vi "move_to.vi"(2 "error in (no error)":errorcluster caption="错误输入（无错误）", 3 "init? (T)":bool=TRUE, 4 "target pos":dbl, 5 "OneMotion 输入":refnum<class "OneMotion.lvclass">) -> (0 "error out":errorcluster caption="错误输出", 1 "OneMotion 输出":refnum<class "OneMotion.lvclass">)   [LabVIEW 2016, in "MotionControl_UFO_3DOF.lvlib" / "OneMotion.lvclass"]
uses:
  <userlib>/MotionControl_UFO_3DOF/OneMotion/OneMotion.lvclass
  <userlib>/MotionControl_UFO_3DOF/OneMotion/OneMotion.lvclass/OneMotion.ctl
  <userlib>/MotionControl_UFO_3DOF/OneMotion/cmd_motion.ctl
  <userlib>/MotionControl_UFO_3DOF/StepMotor/StepMotor.lvclass
  <userlib>/MotionControl_UFO_3DOF/MotionControl_UFO_3DOF.lvlib
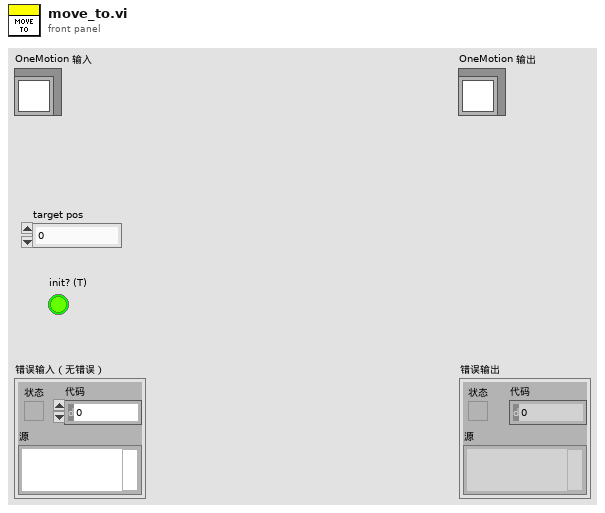
[diagram p1: front panel]
types:
  T1 = cluster{"CAN node ID":i32, "target pos":dbl, "name":string}
  T2 = typedef "MotionControl_UFO_3DOF.lvlib/OneMotion.lvclass/cmd_motion.ctl" = enum16{"NONE", "MOVE_MOTION", "EXIT", "STP_MOTION", "SPEED_MOTION", "WAIT_FOR_S3", "WAIT_A_TIME", "SKIP", "RETRACT_BEFORE_ROT"}
  T3 = cluster{"cmd":T2, cluster{"CAN node ID":i32, "target pos":dbl, "name":string}}
  T4 = cluster{"cmd":T2, cluster{"CAN node ID":i32, "target pos":dbl, "name":string}}[]
  T5 = typedef "MotionControl_UFO_3DOF.lvlib/OneMotion.lvclass/backlash option.ctl" = enum16{"no backlash compensation", "compensation: from - to +", "compensation: from + to -"}
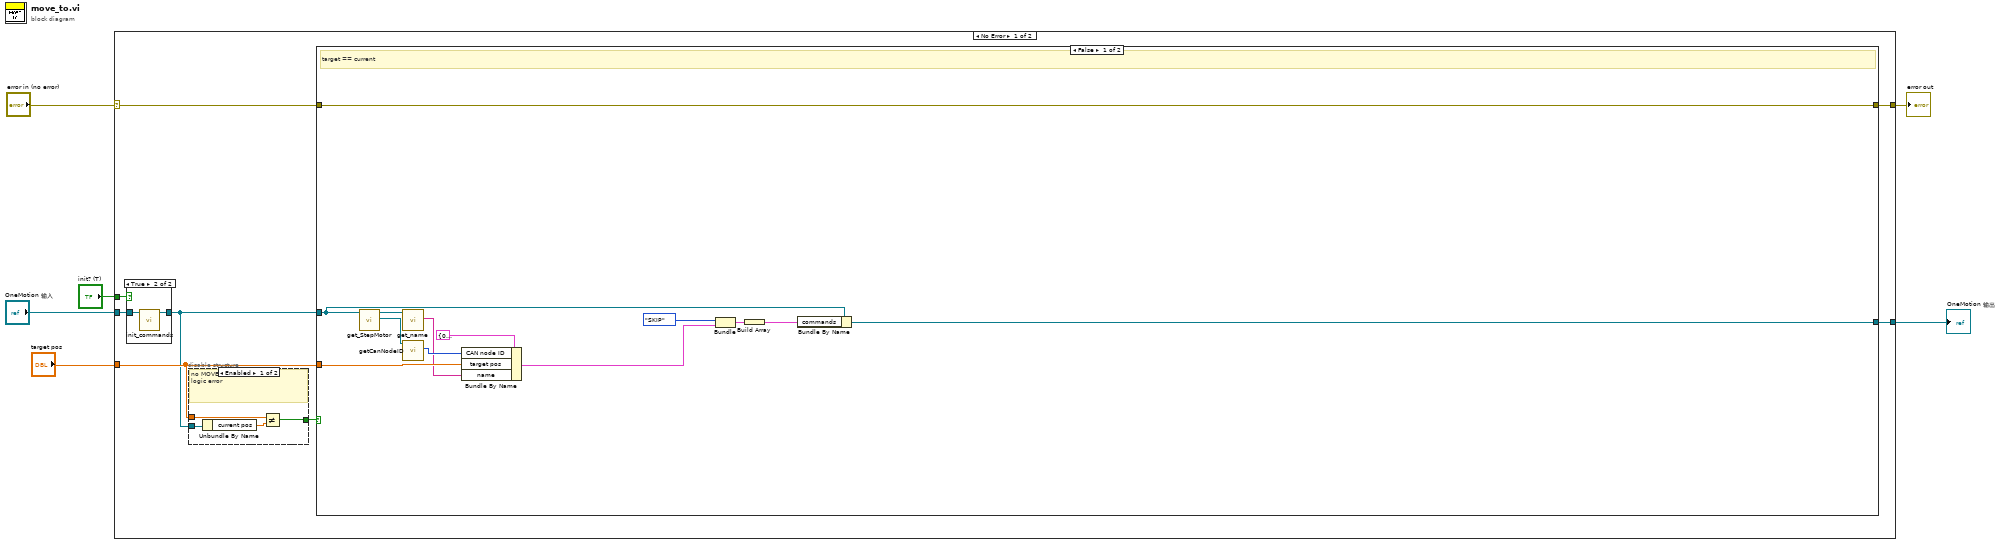
[diagram p0: block diagram]
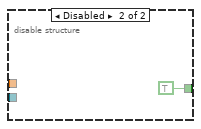
[diagram p2: hidden frame]
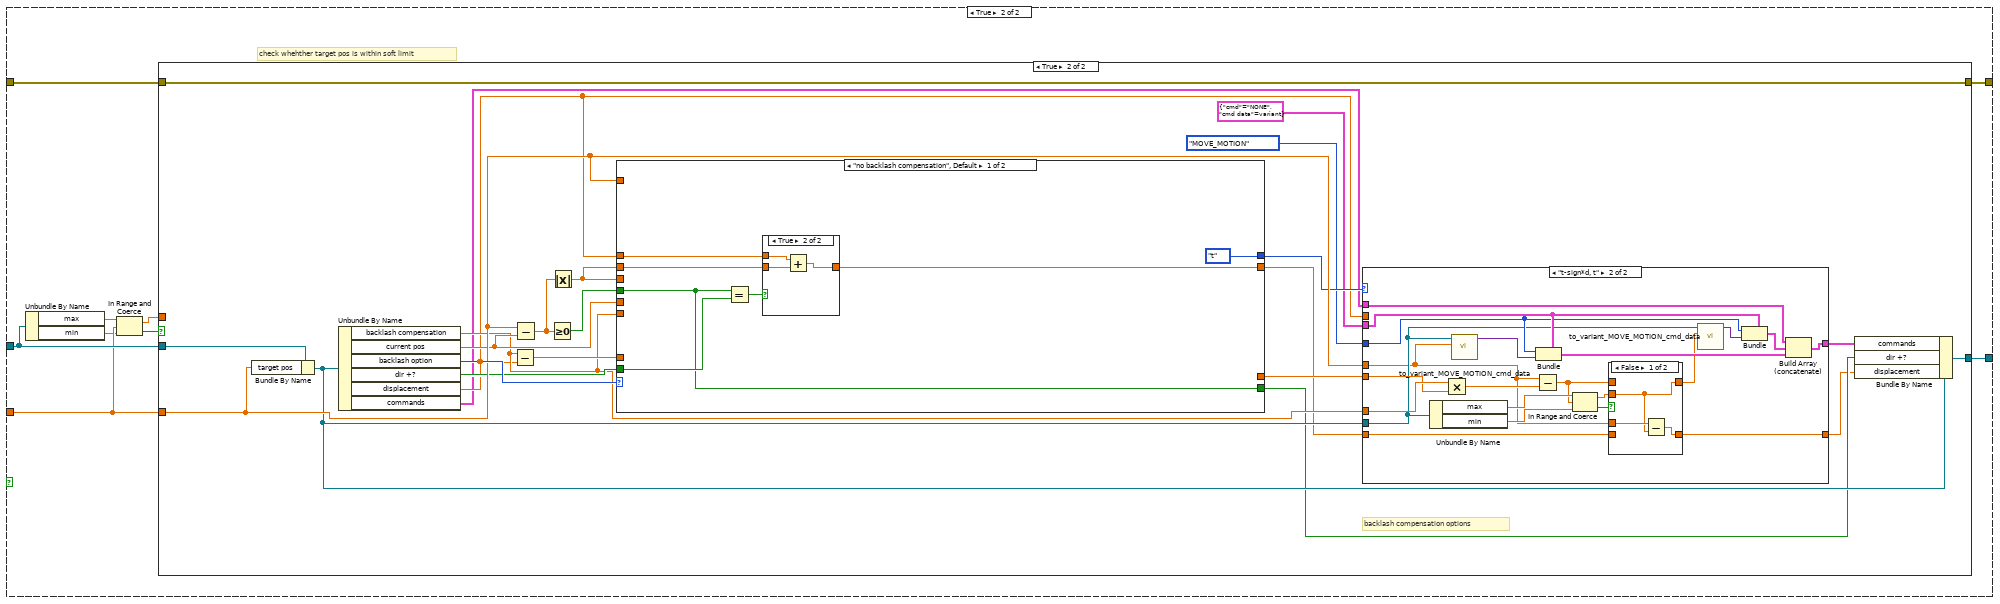
[diagram p4: hidden frame]
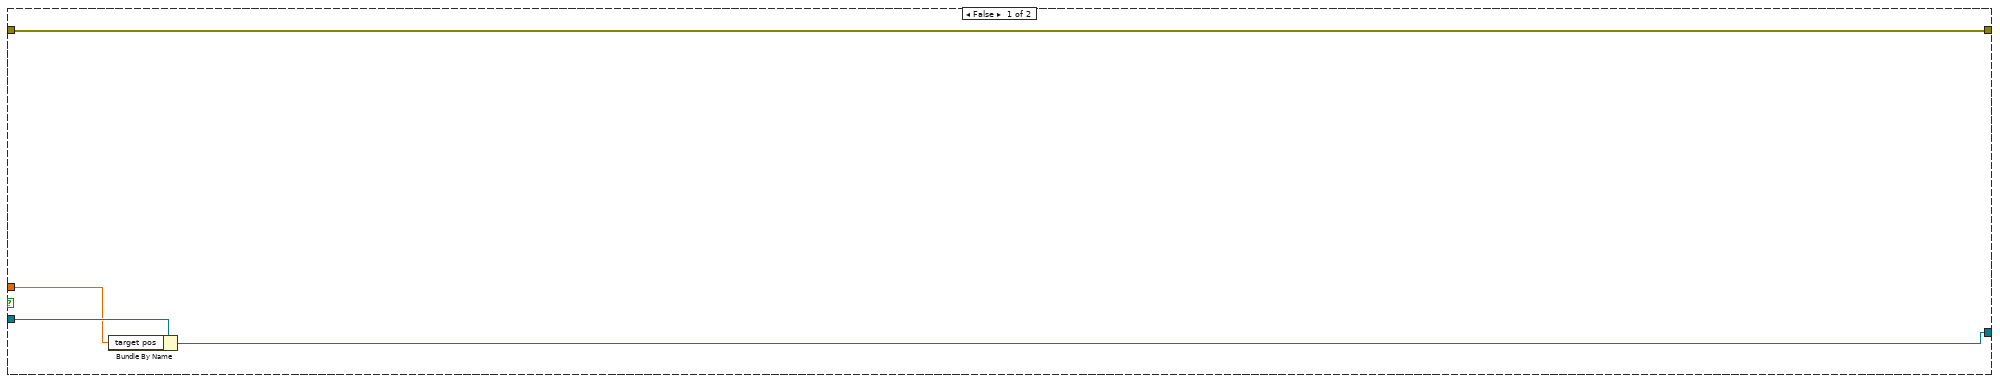
[diagram p5: hidden frame]
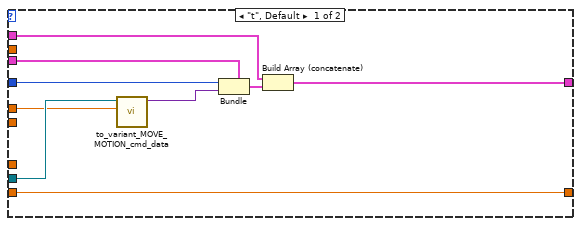
[diagram p6: hidden frame]
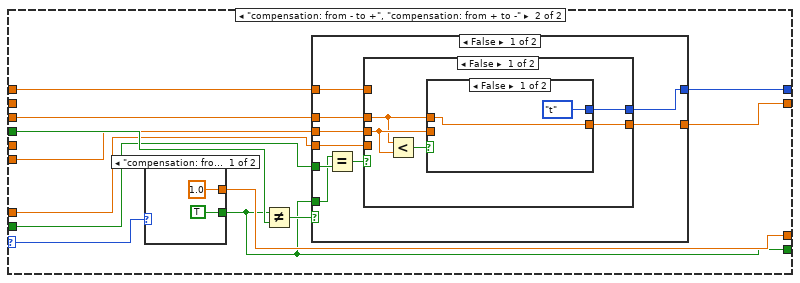
[diagram p9: hidden frame]
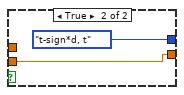
[diagram p10: hidden frame]
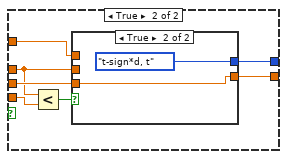
[diagram p11: hidden frame]
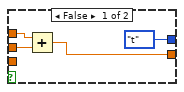
[diagram p12: hidden frame]
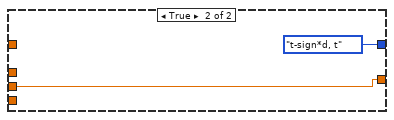
[diagram p13: hidden frame]
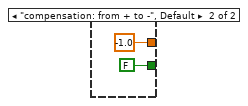
[diagram p14: hidden frame]
diagram:
  n1 = case shown="No Error" "error in (no error)" {
    selector: "error in (no error)" -> [w13 w168]
    tunnel: [w12 w168] -> w5
    tunnel: [w14 w167] -> w4
    tunnel: "OneMotion 输入" -> [w8 w167]
    tunnel: "target pos" -> [w11 _]
    tunnel: "init? (T)" -> [w9 _]
    frame No Error {
      n2 = case shown="True" w9 {
        tunnel: w8 -> [w20 w22]
        tunnel: [w20 w21] -> w7
        frame False {
        }
        frame True {
          n3 = call-dynamic "init_commands.vi"("OneMotion 输入"=w22) -> ("OneMotion 输出"=w21:refnum<class "OneMotion.lvclass">)  [unwired: 9 in, 1 out]
        }
      }
      n4 = disable-structure shown="Enabled" {
        disable-tunnel: w11 -> [w18 _]
        disable-tunnel: [w16 TRUE] -> w10
        disable-tunnel: w7 -> [w15 _]
        frame Enabled {
          # "no MOVE_DONE msg\nlogic error"
          n5 = Unbundle By Name(w15) -> ("current pos"=w17:dbl)
          n6 = Not Equal?(x=w18, y=w17) -> (x != y?=w16:bool)
        }
        frame Disabled {
        }
      }
      n7 = case shown="False" w10 {
        tunnel: [w34 w41] -> w14
        tunnel: w13 -> [w35 w40]
        tunnel: [w35 w39] -> w12
        tunnel: w7 -> [w32 w38]
        tunnel: w11 -> [w27 w37]
        frame False {
          # "target == current"
          n8 = call <userlib>:"get_StepMotor.vi"("OneMotion输入"=w32) -> ("StepMotor.lvclass"=w31:refnum<class "StepMotor.lvclass">, "OneMotion输出"=w24:refnum<class "OneMotion.lvclass">)  [unwired: 8 in, 1 out]
          n9 = call-dynamic "get_name.vi"("OneMotion输入"=w24) -> ("name"=w23:string)  [unwired: 8 in, 2 out]
          n10 = call-dynamic "getCanNodeID.vi"("StepMotor输入"=w31) -> ("CAN node ID"=w28:u32)  [unwired: 8 in, 2 out]
          n11 = Bundle By Name(cluster=T1 {"CAN node ID"=0, "target pos"=0.0, "name"=""}, "CAN node ID"=w28, "target pos"=w27, "name"=w23) -> (w26:T1)
          n12 = Bundle("cmd"=cmd_motion."SKIP", w26) -> (w29:T3)  [unwired: 1 in]
          n13 = Build Array(w29) -> (w33:T4)
          n14 = Bundle By Name(cluster=w32, "commands"=w33) -> (w34:refnum<class "OneMotion.lvclass">)
        }
        frame True {
          # "check whehther target pos is within soft limit"
          n15 = Unbundle By Name(w38) -> ("max"=w44:dbl, "min"=w36:dbl)
          n16 = In Range and Coerce(upper limit=w44, x=w37, lower limit=w36) -> (coerced(x)=w42:dbl, In Range?=w43:bool)
          n17 = case shown="True" w43 {
            tunnel: w38 -> [w48 w70]
            tunnel: w42 -> [w47 _]
            tunnel: [w46 w65] -> w41
            tunnel: w37 -> [_ w69]
            tunnel: w40 -> [w45 w61]
            tunnel: [w45 w61] -> w39
            frame False {
              n18 = Bundle By Name(cluster=w48, "target pos"=w47) -> (w46:refnum<class "OneMotion.lvclass">)
            }
            frame True {
              # "backlash compensation options"
              n19 = Bundle By Name(cluster=w70, "target pos"=w69) -> (w57:refnum<class "OneMotion.lvclass">)
              n20 = Unbundle By Name(w57) -> ("backlash compensation"=w56:dbl, "current pos"=w68:dbl, "backlash option"=w71:T5, "dir +?"=w63:bool, "displacement"=w53:dbl, "commands"=w49:cluster{"cmd":T2, "cmd data":variant}[])
              n21 = Subtract(x=w56, y=w53) -> (x-y=w62:dbl)
              n22 = Subtract(x=w69, y=w68) -> (x-y=w67:dbl)
              n23 = Greater Or Equal To 0?(x=w67) -> (x >= 0?=w64:bool)
              n24 = Absolute Value(x=w67) -> (abs(x)=w54:dbl)
              n25 = case shown="\"no backlash compensation\", Default" w71 {
                selector: w71 -> [_ w129]
                tunnel: w56 -> [_ w122]
                tunnel: w69 -> [_ _]
                tunnel: w68 -> [_ _]
                tunnel: [enum16{"t", "t-sign*d, t"}."t" w126] -> w66
                tunnel: w64 -> [w110 w127]
                tunnel: w63 -> [w112 w125]
                tunnel: w54 -> [_ w124]
                tunnel: w62 -> [_ w123]
                tunnel: [_ w121] -> w55
                tunnel: [w110 w120] -> w52
                tunnel: [w109 w119] -> w51
                tunnel: w54 -> [w108 _]
                tunnel: w53 -> [w107 w118]
                frame "no backlash compensation", Default {
                  n26 = Equal?(x=w110, y=w112) -> (x = y?=w111:bool)
                  n27 = case shown="True" w111 {
                    tunnel: [w114 w117] -> w109
                    tunnel: w108 -> [w114 w116]
                    tunnel: w107 -> [_ w115]
                    frame False {
                    }
                    frame True {
                      n28 = Add(x=w115, y=w116) -> (x+y=w117:dbl)
                    }
                  }
                }
                frame "compensation: from - to +", "compensation: from + to -" {
                  n29 = case shown="\"compensation: from - to +\"" w129 {
                    tunnel: [1.0 -1.0] -> w121
                    tunnel: [TRUE FALSE] -> w120
                    frame "compensation: from - to +" {
                    }
                    frame "compensation: from + to -", Default {
                    }
                  }
                  n30 = Not Equal?(x=w120, y=w127) -> (x != y?=w128:bool)
                  n31 = case shown="False" w128 {
                    tunnel: [w133 enum16{"t", "t-sign*d, t"}."t-sign*d, t"] -> w126
                    tunnel: w125 -> [w137 _]
                    tunnel: w120 -> [w136 _]
                    tunnel: w124 -> [w135 _]
                    tunnel: w123 -> [w134 _]
                    tunnel: w122 -> [w132 w161]
                    tunnel: [w131 w161] -> w119
                    tunnel: w118 -> [w130 _]
                    frame False {
                      n32 = Equal?(x=w136, y=w137) -> (x = y?=w138:bool)
                      n33 = case shown="False" w138 {
                        tunnel: w135 -> [w139 w148]
                        tunnel: w134 -> [_ w153]
                        tunnel: [w142 w152] -> w133
                        tunnel: w132 -> [w141 w151]
                        tunnel: [w140 w150] -> w131
                        tunnel: w130 -> [_ w149]
                        frame False {
                          n34 = Less?(x=w139, y=w141) -> (x < y?=w143:bool)
                          n35 = case shown="False" w143 {
                            tunnel: [enum16{"t", "t-sign*d, t"}."t" enum16{"t", "t-sign*d, t"}."t-sign*d, t"] -> w142
                            tunnel: w141 -> [_ w146]
                            tunnel: [w144 w146] -> w140
                            tunnel: w139 -> [w144 _]
                            frame False {
                            }
                            frame True {
                            }
                          }
                        }
                        frame True {
                          n36 = Less?(x=w148, y=w153) -> (x < y?=w154:bool)
                          n37 = case shown="True" w154 {
                            tunnel: [enum16{"t", "t-sign*d, t"}."t" enum16{"t", "t-sign*d, t"}."t-sign*d, t"] -> w152
                            tunnel: w151 -> [_ w159]
                            tunnel: [w155 w159] -> w150
                            tunnel: w149 -> [w157 _]
                            tunnel: w148 -> [w156 _]
                            frame False {
                              n38 = Add(x=w157, y=w156) -> (x+y=w155:dbl)
                            }
                            frame True {
                            }
                          }
                        }
                      }
                    }
                    frame True {
                    }
                  }
                }
              }
              n39 = case shown="\"t-sign*d, t\"" w66 {
                tunnel: w57 -> [w78 w89]
                tunnel: w69 -> [w77 w84]
                tunnel: [w76 w99] -> w60
                tunnel: cluster{"cmd":T2, "cmd data":variant} {"cmd"=enum."NONE", "cmd data"=variant} ("command cluster") -> [w75 w97]
                tunnel: cmd_motion."MOVE_MOTION" ("cmd") -> [w74 w96]
                tunnel: w56 -> [_ w94]
                tunnel: w55 -> [_ w93]
                tunnel: w53 -> [_ _]
                tunnel: [w73 w83] -> w50
                tunnel: w51 -> [w73 w82]
                tunnel: w49 -> [w72 w81]
                frame "t", Default {
                  n40 = call <userlib>:"to_variant_MOVE_MOTION_cmd_data.vi"("target pos"=w77, "OneMotion.lvclass"=w78) -> ("variant"=w80:variant)  [unwired: 9 in]
                  n41 = Bundle(cluster=w75, "cmd"=w74, "cmd data"=w80) -> (w79:cluster{"cmd":T2, "cmd data":variant})
                  n42 = Build Array (concatenate)(w72, w79) -> (w76:cluster{"cmd":T2, "cmd data":variant}[])
                }
                frame "t-sign*d, t" {
                  n43 = Unbundle By Name(w89) -> ("max"=w91:dbl, "min"=w90:dbl)
                  n44 = Multiply(x=w94, y=w93) -> (x*y=w92:dbl)
                  n45 = call <userlib>:"to_variant_MOVE_MOTION_cmd_data.vi"("target pos"=w84, "OneMotion.lvclass"=w89) -> ("variant"=w101:variant)  [unwired: 9 in]
                  n46 = Subtract(x=w84, y=w92) -> (x-y=w86:dbl)
                  n47 = Bundle(cluster=w97, "cmd"=w96, "cmd data"=w101) -> (w100:cluster{"cmd":T2, "cmd data":variant})
                  n48 = In Range and Coerce(upper limit=w91, x=w86, lower limit=w90) -> (coerced(x)=w87:dbl, In Range?=w88:bool)
                  n49 = case shown="False" w88 {
                    tunnel: w87 -> [w103 _]
                    tunnel: w86 -> [_ w106]
                    tunnel: [w103 w106] -> w85
                    tunnel: w84 -> [w104 _]
                    tunnel: [w102 w105] -> w83
                    tunnel: w82 -> [_ w105]
                    frame False {
                      n50 = Subtract(x=w104, y=w103) -> (x-y=w102:dbl)
                    }
                    frame True {
                    }
                  }
                  n51 = call <userlib>:"to_variant_MOVE_MOTION_cmd_data.vi"("target pos"=w85, "OneMotion.lvclass"=w89) -> ("variant"=w98:variant)  [unwired: 9 in]
                  n52 = Bundle(cluster=w97, "cmd"=w96, "cmd data"=w98) -> (w95:cluster{"cmd":T2, "cmd data":variant})
                  n53 = Build Array (concatenate)(w81, w95, w100) -> (w99:cluster{"cmd":T2, "cmd data":variant}[])
                }
              }
              n54 = Bundle By Name(cluster=w57, "commands"=w60, "dir +?"=w52, "displacement"=w50) -> (w65:refnum<class "OneMotion.lvclass">)
            }
          }
        }
      }
    }
    frame Error {
    }
  }
  "error out" <- w5
  "OneMotion 输出" <- w4
